vi "Write Acquisition type.vi"(8 "error in (no error)":errorcluster, 10 "Acquisition type":string(combo), 11 "DAQ Configuration in":refnum<class "DAQ Configuration.lvclass">) -> (0 "error out":errorcluster, 3 "DAQ Configuration out":refnum<class "DAQ Configuration.lvclass">)   [LabVIEW 2026, in "Hardware.lvlib" / "DAQ Configuration.lvclass"]
uses:
  DAQ Configuration.lvclass
  DAQ Configuration.lvclass/DAQ Configuration.ctl
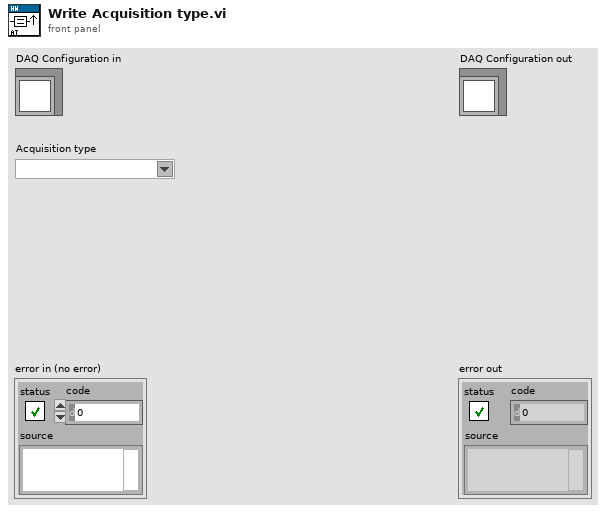
[diagram p1: front panel]
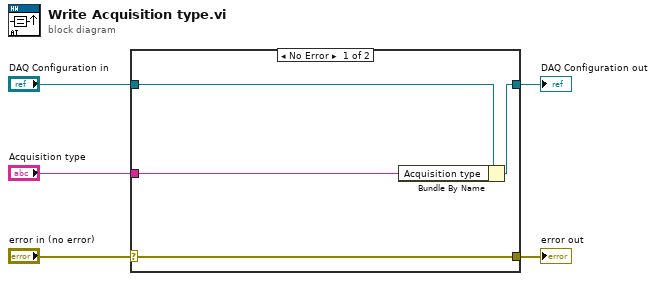
[diagram p0: block diagram]
diagram:
  n1 = case shown="No Error" "error in (no error)" {
    selector: "error in (no error)" -> [w9 w10]
    tunnel: [w9 w10] -> w4
    tunnel: [w7 w11] -> w2
    tunnel: "DAQ Configuration in" -> [w8 w11]
    tunnel: "Acquisition type" -> [w6 _]
    frame No Error {
      n2 = Bundle By Name(cluster=w8, "Acquisition type"=w6) -> (w7:refnum<class "DAQ Configuration.lvclass">)
    }
    frame Error {
    }
  }
  "error out" <- w4
  "DAQ Configuration out" <- w2
